vi "Check Grapes.vi"(7 "Packed refs":T1, 8 "error in (no error)":errorcluster, 11 "Board Game in":refnum<class "Board Game.lvclass">) -> (0 "error out":errorcluster, 3 "Board Game out":refnum<class "Board Game.lvclass">)   [LabVIEW 2021, in "Board Game.lvclass"]
uses:
  Board Game.lvclass
  Application/Packed Refs.ctl
  GameEl_class/private/Enum Direction.ctl
  Board Game.lvclass/Board Game.ctl
  GameEl_class/GameEl.lvclass/GameEl.ctl
  Grape/Grape.lvclass/Grape.ctl
  Snake_class/Snake.lvclass/Snake.ctl
  Imposible_Snake_v2/LVApp/Modules/Sound Manager/Typedefs/Sound Effects.ctl
  <vilib>/numeric/Random Number (Range) U64.vi
  Snake_class/Write Grapes.vi
  Grape/Write Ate timestamp.vi
  Grape/Write ActiveEffect.vi
  GameEl_class/Write Visible.vi
  Snake_class/Read Snake Head.vi
  Snake_class/Read Star.vi
  GameEl_class/Read Visible.vi
  GameEl_class/Read position.vi
  Grape/Read ActiveEffect.vi
  Grape/Read Grapes.vi
  <vilib>/numeric/sub_Random U32.vi
  Grape/Grape.lvclass
  C:/Users/poche/Programs/LabVIEW/imposible snake/GameEl_class/GameEl.lvclass
  Snake_class/Snake.lvclass
  Imposible_Snake_v2/LVApp/Modules/Sound Manager/Sound Manager.lvlib
  GameEl_class/GameEl.lvclass
  Application/Game.lvclass
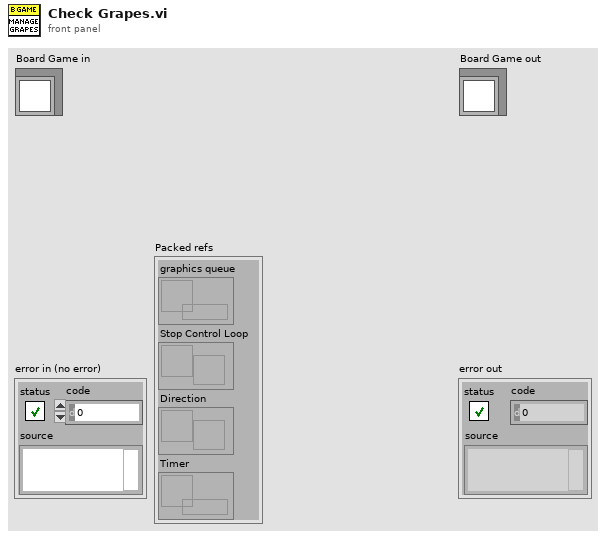
[diagram p1: front panel]
types:
  T1 = typedef "Game.lvclass/Packed Refs.ctl" = cluster{"graphics queue":refnum<queue>, "Stop Control Loop":refnum<user-event>, "Direction":refnum<notifier>, "Timer":refnum<data-value>}
  T2 = typedef "Sound Manager.lvlib/Sound Effects.ctl" = enum16{"Bomb In", "Bomb Out", "Bomb Touched", "Game Over", "Victory", "Eat", "10 Fruits", "Eat2", "Eat3", "Eat4", "MaxShield", "Shield", "10p", "Grape In", "Grape Out", "20p", "30p", "40p", "50p", "60p", "70p", "80p", "90p", "100p", "All shields cracked", "Mouse In", "Mouse Out", "Mouse Eaten", "Grape Eaten", "States Recover", "Broken Shield", "Bonus", "Happy Time", "explode", "Game over musica", "Back Music", "Shield Catch", "Evil lough", "Cricket In", "Cricket eaten", "Lets Go", "Jump1", "Jump2", "Jump3", "Unstoppable", "Troll Music", "winner", "menu"}
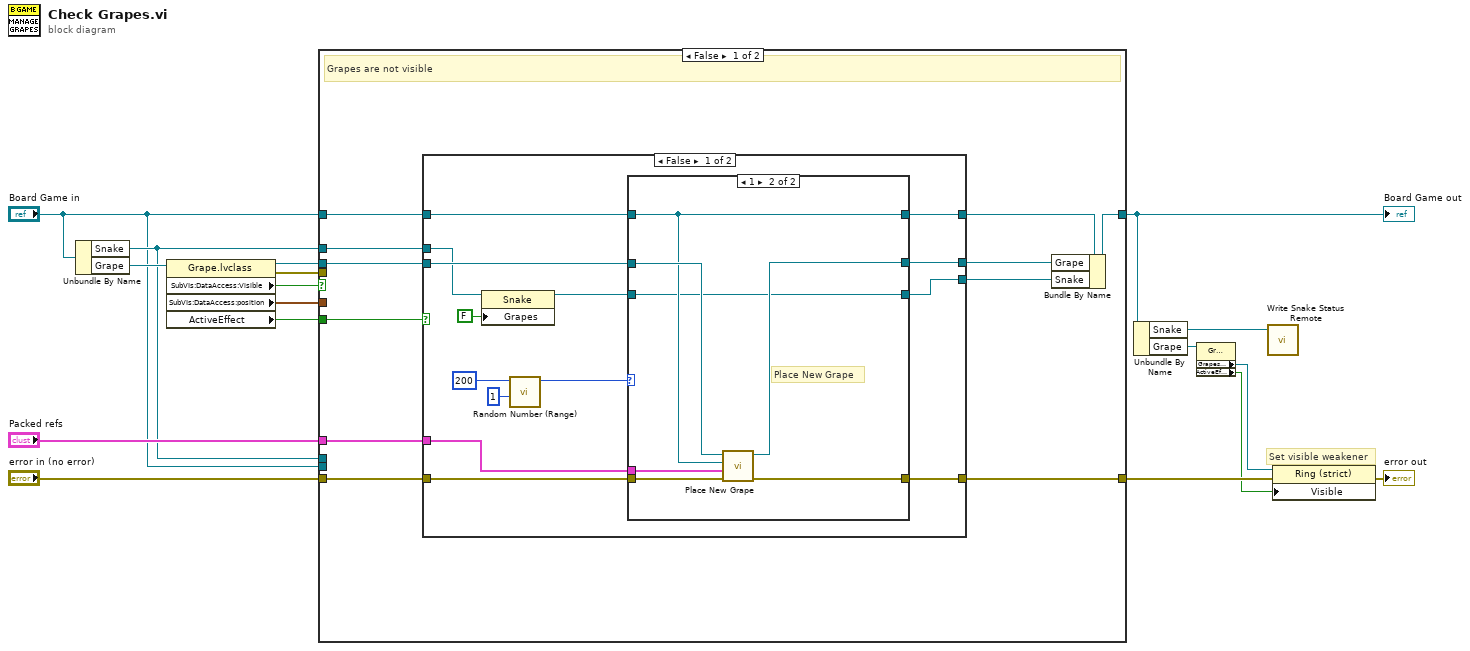
[diagram p0: block diagram]
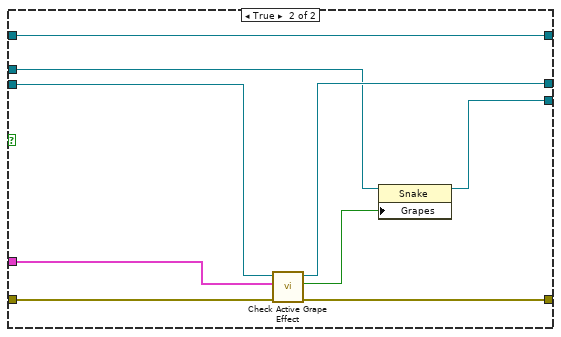
[diagram p3: hidden frame]
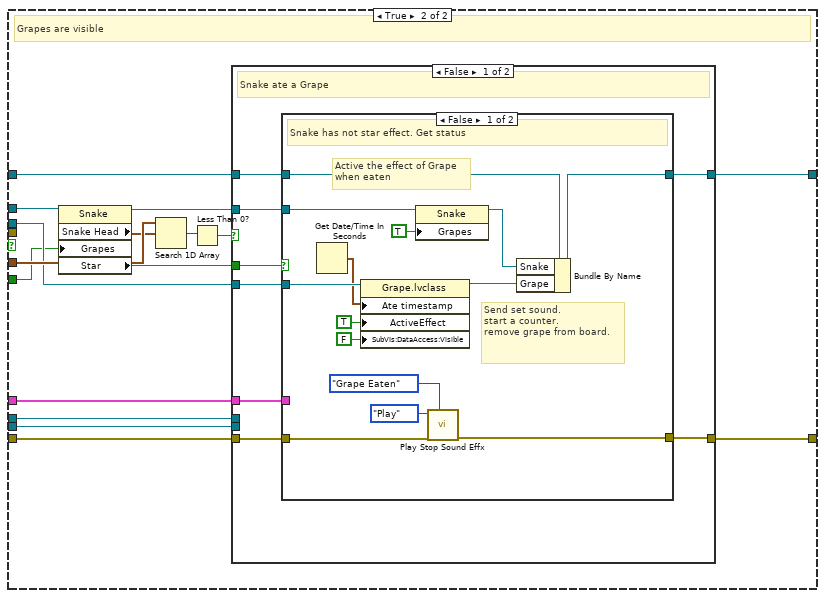
[diagram p4: hidden frame]
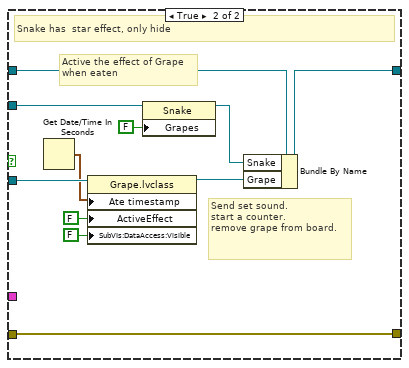
[diagram p5: hidden frame]
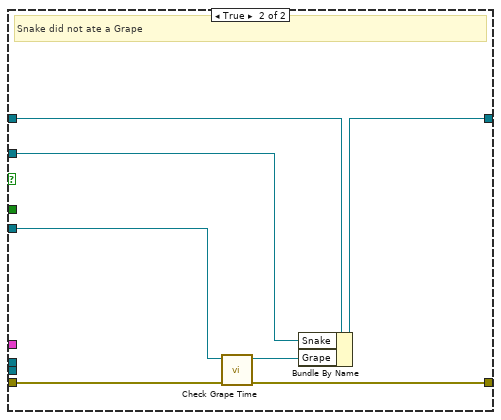
[diagram p6: hidden frame]
diagram:
  # "Set visible weakener"
  n1 = Unbundle By Name("Board Game in") -> ("Snake"=w2:refnum<class "Snake.lvclass">, "Grape"=w17:refnum<class "Grape.lvclass">)
  n2 = property class="Grape.lvclass"(reference=w17) -> (reference out=w14:refnum<class "Grape.lvclass">, error out=w12:errorcluster, "SubVIs:DataAccess:Visible"=w15:bool, "SubVIs:DataAccess:position"=w13:cluster{"x":dbl, "y":dbl}[], "ActiveEffect"=w11:bool)  [unwired: 1 in]
  n3 = case shown="False" w15 {
    tunnel: "error in (no error)" -> [w26 w74]
    tunnel: "Board Game in" -> [w28 w72]
    tunnel: [w23 w71] -> w8
    tunnel: [w25 w73] -> w10
    tunnel: w14 -> [w24 w69]
    tunnel: w2 -> [w20 w78]
    tunnel: w13 -> [_ w77]
    tunnel: w12 -> [_ _]
    tunnel: w11 -> [w21 w68]
    tunnel: "Packed refs" -> [w18 w66]
    tunnel: w2 -> [_ w65]
    tunnel: "Board Game in" -> [_ w64]
    frame False {
      # "Grapes are not visible"
      n4 = case shown="False" w21 {
        tunnel: w28 -> [w40 w62]
        tunnel: [w39 w62] -> w27
        tunnel: w26 -> [w37 w60]
        tunnel: [w36 w59] -> w25
        tunnel: w24 -> [w35 w61]
        tunnel: [w34 w58] -> w22
        tunnel: w20 -> [w33 w57]
        tunnel: [w30 w55] -> w19
        tunnel: w18 -> [w29 w54]
        frame False {
          n5 = property class="Snake"(reference=w33, "Grapes"=FALSE) -> (reference out=w31:refnum<class "Snake.lvclass">)  [unwired: 1 in, 1 out]
          n6 = call-poly <vilib>:"Random Number (Range).vi"("lower bound (0)"=u64 1, "upper bound (100)"=u64 200) -> ("number"=w38:u64)  [unwired: 9 in]
          n7 = case shown="1" w38 {
            tunnel: w40 -> [w46 w49]
            tunnel: [w46 w49] -> w39
            tunnel: w37 -> [w45 w53]
            tunnel: [w45 w50] -> w36
            tunnel: w35 -> [w44 w52]
            tunnel: [w44 w51] -> w34
            tunnel: w31 -> [w43 w48]
            tunnel: [w43 w48] -> w30
            tunnel: w29 -> [_ w47]
            frame 0, Default {
            }
            frame 1 {
              # "Place New Grape"
              n8 = call "Place New Grape.vi"("error in (no error)"=w53, "Packed refs"=w47, "Board Game in"=w49, "Grape in"=w52) -> ("error out"=w50:errorcluster, "Grape out"=w51:refnum<class "Grape.lvclass">)  [unwired: 6 in]
            }
          }
        }
        frame True {
          n9 = call "Check Active Grape Effect.vi"("error in (no error)"=w60, "Packed refs"=w54, "Grape in"=w61) -> ("error out"=w59:errorcluster, "Still Active?"=w56:bool, "Grape out"=w58:refnum<class "Grape.lvclass">)  [unwired: 6 in]
          n10 = property class="Snake"(reference=w57, "Grapes"=w56) -> (reference out=w55:refnum<class "Snake.lvclass">)  [unwired: 1 in, 1 out]
        }
      }
      n11 = Bundle By Name(cluster=w27, "Grape"=w22, "Snake"=w19) -> (w23:refnum<class "Board Game.lvclass">)
    }
    frame True {
      # "Grapes are visible"
      n12 = property class="Snake"(reference=w78, "Grapes"=w68) -> (reference out=w67:refnum<class "Snake.lvclass">, "Snake Head"=w76:cluster{"x":dbl, "y":dbl}, "Star"=w63:bool)  [unwired: 1 in, 1 out]
      n13 = Search 1D Array(1D array=w77, element=w76) -> (index of element=w75:i32)  [unwired: 1 in]
      n14 = Less Than 0?(x=w75) -> (x < 0?=w70:bool)
      n15 = case shown="False" w70 {
        tunnel: w74 -> [w81 w117]
        tunnel: [w80 w115] -> w73
        tunnel: w72 -> [w86 w118]
        tunnel: [w85 w114] -> w71
        tunnel: w69 -> [w84 w116]
        tunnel: w67 -> [w83 w112]
        tunnel: w66 -> [w82 _]
        tunnel: w65 -> [_ _]
        tunnel: w64 -> [_ _]
        tunnel: w63 -> [w79 _]
        frame False {
          # "Snake ate a Grape"
          n16 = case shown="False" w79 {
            tunnel: w86 -> [w100 w111]
            tunnel: [w99 w110] -> w85
            tunnel: w84 -> [w98 w109]
            tunnel: w83 -> [w93 w104]
            tunnel: w82 -> [_ _]
            tunnel: w81 -> [w88 w101]
            tunnel: [w87 w101] -> w80
            frame False {
              # "Active the effect of Grape\nwhen eaten"
              # "Send set sound.\nstart a counter.\nremove grape from board."
              # "Snake has not star effect. Get status"
              n17 = Get Date/Time In Seconds() -> (seconds since 1Jan1904=w97:timestamp)
              n18 = property class="Grape.lvclass"(reference=w98, "Ate timestamp"=w97, "ActiveEffect"=TRUE, "SubVIs:DataAccess:Visible"=FALSE ("Visible")) -> (reference out=w95:refnum<class "Grape.lvclass">)  [unwired: 1 in, 1 out]
              n19 = property class="Snake"(reference=w93, "Grapes"=TRUE) -> (reference out=w91:refnum<class "Snake.lvclass">)  [unwired: 1 in, 1 out]
              n20 = call "Play Stop Sound Effx.vi"("Sound Effect"=Sound_Effects."Grape Eaten", "Error In"=w88, "Function"=enum16{"Play", "Stop"}."Play") -> ("error in (no error)"=w87:errorcluster)  [unwired: 8 in]
              n21 = Bundle By Name(cluster=w100, "Snake"=w91, "Grape"=w95) -> (w99:refnum<class "Board Game.lvclass">)
            }
            frame True {
              # "Active the effect of Grape\nwhen eaten"
              # "Send set sound.\nstart a counter.\nremove grape from board."
              # "Snake has  star effect, only hide"
              n22 = Get Date/Time In Seconds() -> (seconds since 1Jan1904=w108:timestamp)
              n23 = property class="Grape.lvclass"(reference=w109, "Ate timestamp"=w108, "ActiveEffect"=FALSE, "SubVIs:DataAccess:Visible"=FALSE ("Visible")) -> (reference out=w106:refnum<class "Grape.lvclass">)  [unwired: 1 in, 1 out]
              n24 = property class="Snake"(reference=w104, "Grapes"=FALSE) -> (reference out=w102:refnum<class "Snake.lvclass">)  [unwired: 1 in, 1 out]
              n25 = Bundle By Name(cluster=w111, "Snake"=w102, "Grape"=w106) -> (w110:refnum<class "Board Game.lvclass">)
            }
          }
        }
        frame True {
          # "Snake did not ate a Grape"
          n26 = call "Check Grape Time.vi"("error in (no error)"=w117, "Grape in"=w116) -> ("error out"=w115:errorcluster, "Grape out"=w113:refnum<class "Grape.lvclass">)  [unwired: 8 in]
          n27 = Bundle By Name(cluster=w118, "Snake"=w112, "Grape"=w113) -> (w114:refnum<class "Board Game.lvclass">)
        }
      }
    }
  }
  "Board Game out" <- w8
  n28 = Unbundle By Name(w8) -> ("Snake"=w4:refnum<class "Snake.lvclass">, "Grape"=w7:refnum<class "Grape.lvclass">)
  n29 = property class="Grape.lvclass"(reference=w7) -> ("Grapes Ref"=w6:refnum<vi>, "ActiveEffect"=w5:bool)  [unwired: 1 in, 2 out]
  n30 = call "Write Snake Status Remote.vi"("Snake in"=w4) -> ()  [unwired: 9 in, 2 out]
  n31 = property class="Ring (strict)"(reference=w6, error in=w10, "Visible"=w5) -> (error out=→"error out":errorcluster)  [unwired: 1 out]
